vi "Close File.vi"(8 "error in":errorcluster, 11 "File in":refnum<file>) -> (0 "error out":errorcluster)   [LabVIEW 2017]
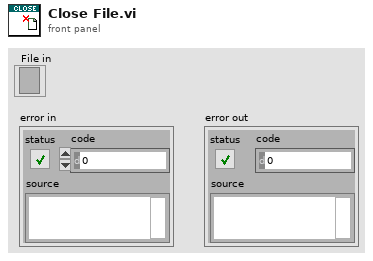
[diagram p1: front panel]
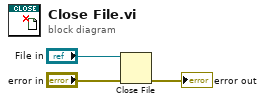
[diagram p0: block diagram]
diagram:
  n1 = Close File(refnum="File in", error in="error in") -> (error out=→"error out":errorcluster)  [unwired: 1 out]
